vi "VirtualKeyboard.vi"(7 "eShiftMode":enum8{"Up", "Down"}(ring), 8 "error in (no error)":errorcluster, 11 "eKey":u16(ring)=16 items=["NONE", "LBUTTON", "RBUTTON", "CANCEL", "MBUTTON", "XBUTTON1", "XBUTTON2", "NONE", "BACKSPACE", "TAB", "NONE", "NONE", "CLEAR", "ENTER", "NONE", "NONE", "SHIFT", "CTRL", "ALT", "PAUSE", "CAPSLOCK", "KANA", "HANGUL", "JUNJA", "FINAL", "HANJA", "KANJI", "ESC", "CONVERT", "NONCONVERT", "ACCEPT", "MODECHANGE", "SPACE", "PAGEUP", "PAGEDOWN", "END", "HOME", "LEFT", "UP", "RIGHT", "DOWN", "SELECT", "PRINT", "EXECUTE", "SNAPSHOT", "INSERT", "DELETE", "HELP", "0", "1", "2", "3", "4", "5", "6", "7", "8", "9", "NONE", "NONE", "NONE", "NONE", "NONE", "NONE", "NONE", "A", "B", "C", "D", "E", "F", "G", "H", "I", "J", "K", "L", "M", "N", "O", "P", "Q", "R", "S", "T", "U", "V", "W", "X", "Y", "Z", "LWIN", "RWIN", "APPS", "NONE", "SLEEP", "NUMPAD0", "NUMPAD1", "NUMPAD2", "NUMPAD3", "NUMPAD4", "NUMPAD5", "NUMPAD6", "NUMPAD7", "NUMPAD8", "NUMPAD9", "MULTIPLE", "ADD", "SEPARATOR", "SUBSTRACT", "DECIMAL", "DIVIDE", "F1", "F2", "F3", "F4", "F5", "F6", "F7", "F8", "F9", "F10", "F11", "F12", "F13", "F14", "F15", "F16", "F17", "F18", "F19", "F20", "F21", "F22", "F23", "F24", "NONE", "NONE", "NONE", "NONE", "NONE", "NONE", "NONE", "NONE", "NUMLOCK", "SCROLL", "NONE", "NONE", "NONE", "NONE", "NONE", "NONE", "NONE", "NONE", "NONE", "NONE", "NONE", "NONE", "NONE", "NONE", "LSHIFT", "RSHIFT", "LCONTROL", "RCONTROL", "LMENU", "RMENU", "BROWSER_BACK", "BROWSER_FORWARD", "BROWSER_REFRESH", "BROWSER_STOP", "BROWSER_SEARCH", "BROWSER _FAVORITES", "BROWSER_HOME", "VOLUME_MUTE", "VOLUME_DOWN", "VOLUME_UP", "MEDIA_NEXT_TRACK", "MEDIA_PREV_TRACK", "MEDIA_STOP", "MEDIA_PLAY_PAUSE", "LAUNCH_MAIL", "LAUNCH_MEDIA_SELECT", "LAUNCH_APP1", "LAUNCH_APP2", "NONE", "NONE", ";:", "=+", ",<", "-_", ".>", "/?", "`~", "NONE", "NONE", "NONE", "NONE", "NONE", "NONE", "NONE", "NONE", "NONE", "NONE", "NONE", "NONE", "NONE", "NONE", "NONE", "NONE", "NONE", "NONE", "NONE", "NONE", "NONE", "NONE", "NONE", "NONE", "NONE", "NONE", "[{", "\\|", "]}", "'\""]) -> (0 "error out":errorcluster)   [LabVIEW 2017]
doc: "功能：\n虚拟键盘，可虚拟实现各个按键的“按下”、“弹起”功能"
uses:
  user32.dll
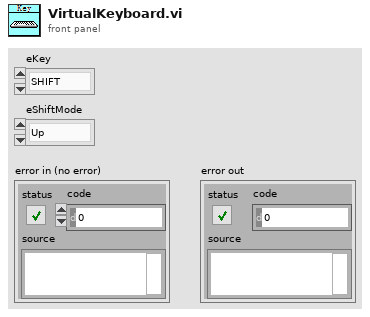
[diagram p1: front panel]
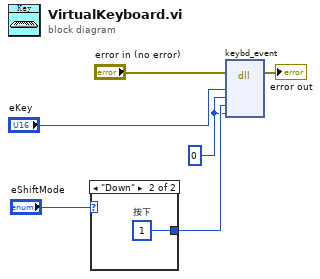
[diagram p0: block diagram]
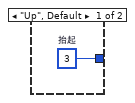
[diagram p2: hidden frame]
diagram:
  w2 = 0 ("bScan")
  n1 = case shown="\"Down\"" "eShiftMode" {
    tunnel: [w7 w8] -> w4
    frame "Up", Default {
      w7 = 3  # 抬起
    }
    frame "Down" {
      w8 = 1  # 按下
    }
  }
  n2 = dll-call lib="user32.dll" fn="keybd_event"(error in="error in (no error)", "bVK"="eKey", "bScan"=w2, "dwFlags"=w4, "dwExtraInfo"=w2) -> (error out=→"error out":errorcluster)  [unwired: 7 in, 1 out]
